vi "Locate HPRF Spark Laterally.vi"(5 "Ntheta":i32=16, 6 "Sensor Locations (cm)":dbl[][](array[numeric])=[[0.0, 0.0, -5.08], [11.43, 0.0, 0.0], [0.0, 11.43, 0.0], [-11.43, 0.0, 0.0], [0.0, -11.43, 0.0], [0.0, 0.0, 5.08]], 7 "Nr":i32=16, 8 "Sound Velocity (cm/s)":dbl=576000.0, 9 "Sampling Rate":i32=500000, 11 "Waveforms":dbl[][](array[numeric])) -> (2 "Coordinates (m)":cluster{"x":dbl, "y":dbl})   [LabVIEW 2013]
uses:
  <vilib>/Analysis/2dsp.llb/1D Cross Correlation (DBL).vi
  <vilib>/Analysis/NI_AALPro.lvlib
panel:
  out "Signals":dbl[][](graph)
  out "output variable 3":dbl
  out "output variable 2":dbl
  out "output variable":dbl
  out "subarray":dbl[][](array[numeric])
  out "size(s)":i32[](array[numeric])
  out "theta":dbl
  out "r":dbl
  out "Correlation":dbl[][](graph)
  out "Lag Matrix":dbl[][](array[numeric])
  # "Inputs"
  # "Output"
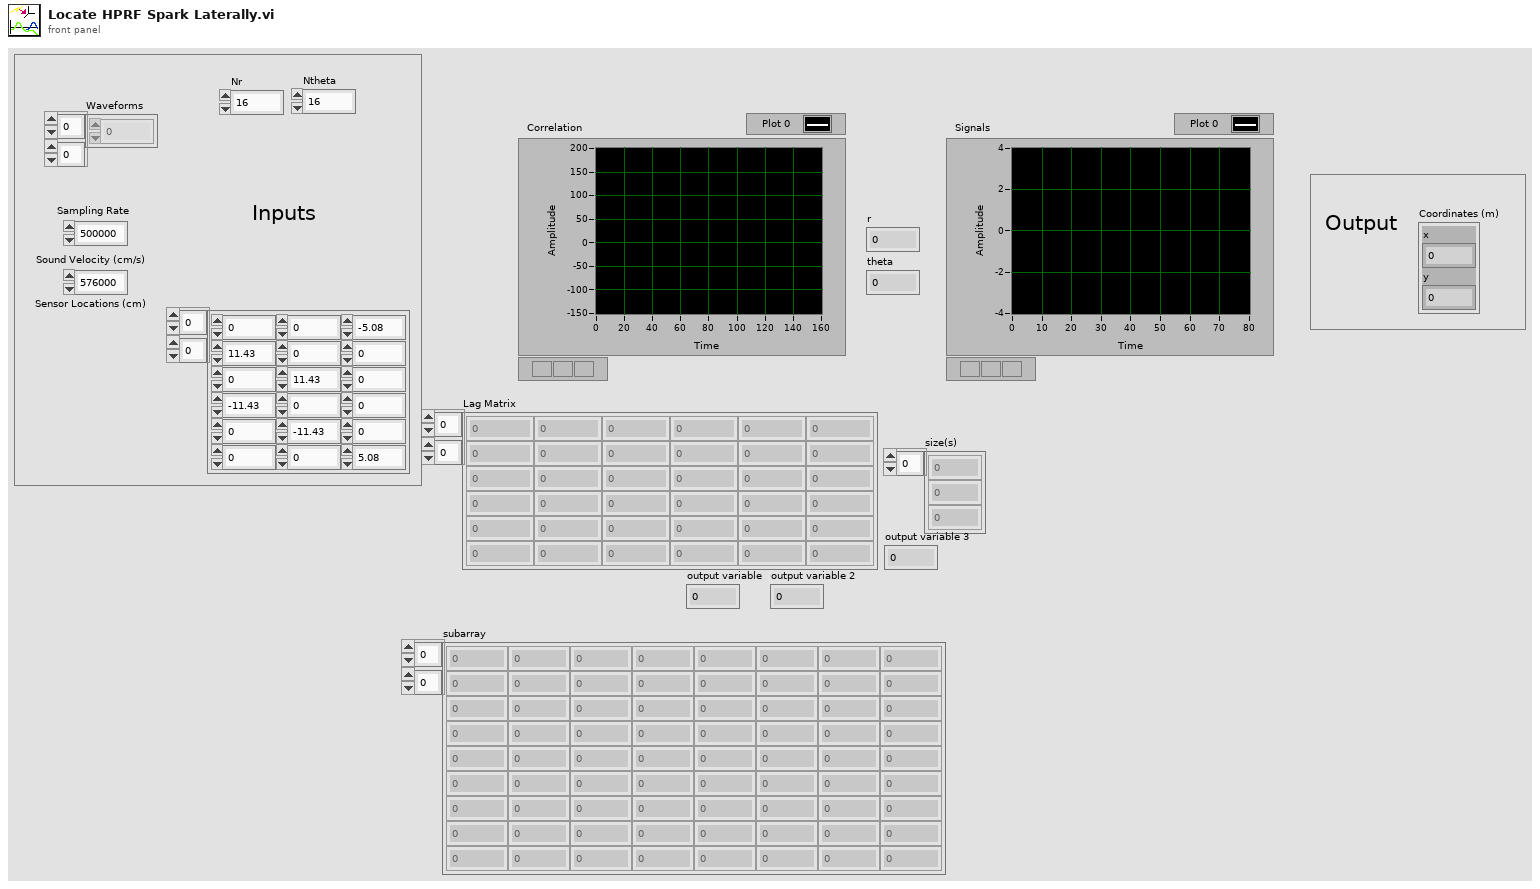
[diagram p1: front panel]
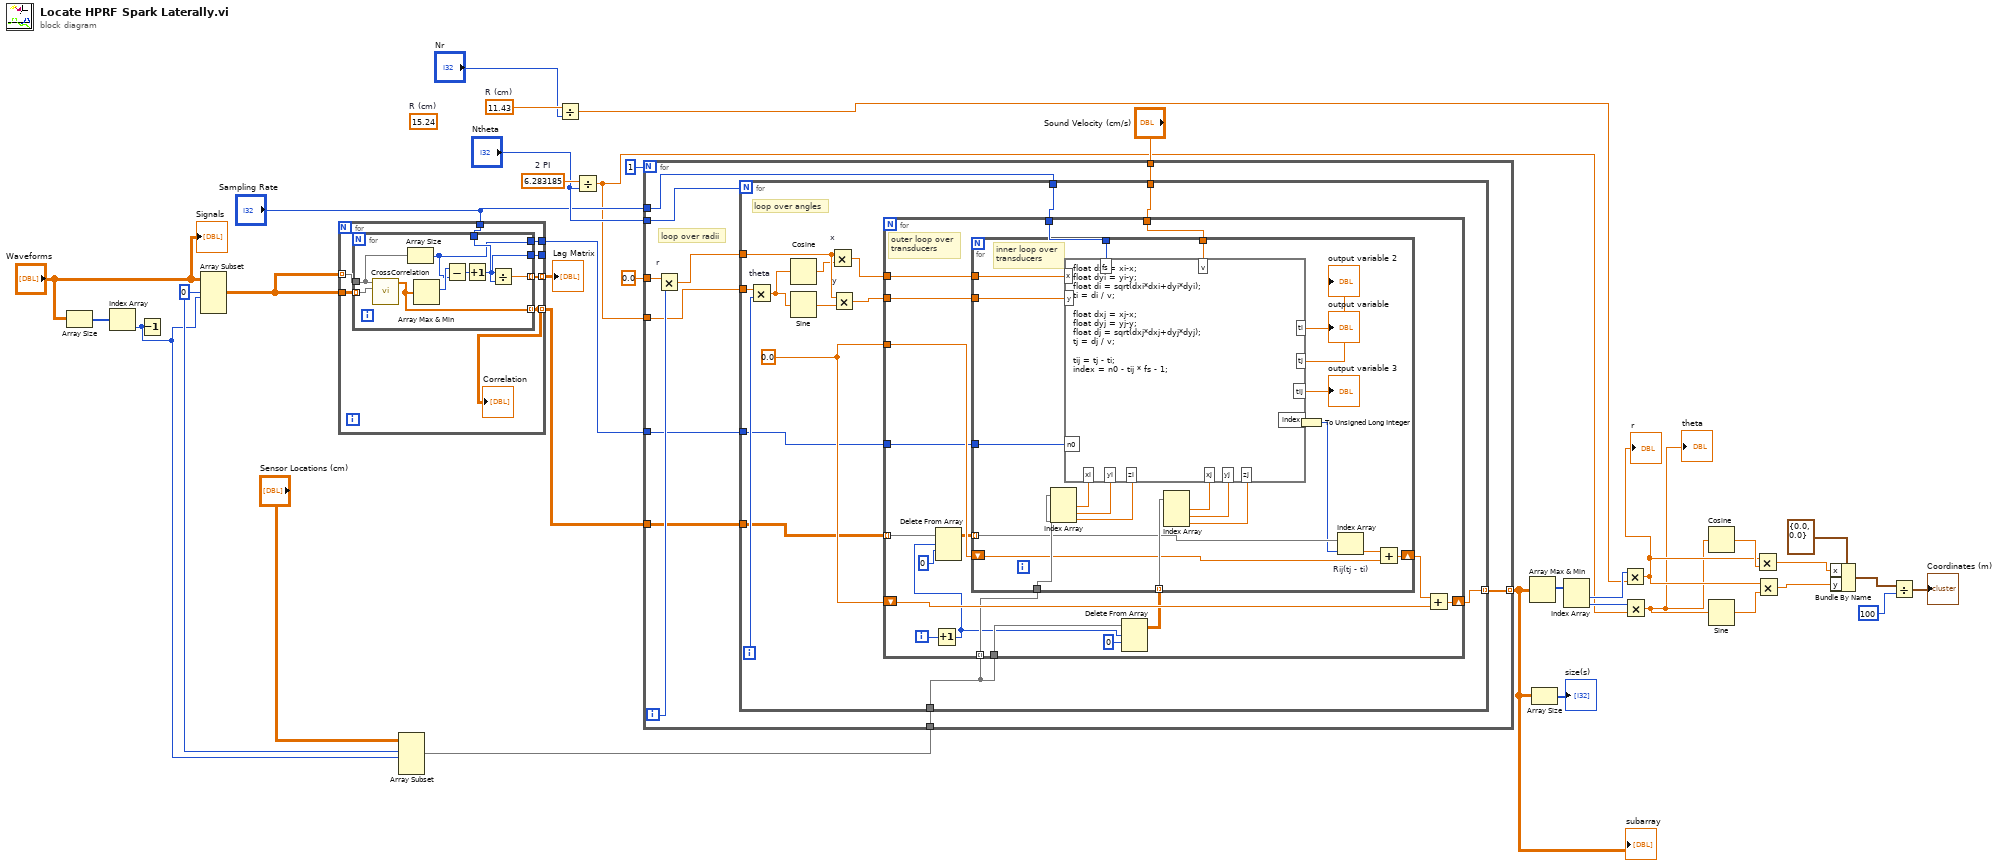
[diagram p0: block diagram]
diagram:
  (unwired) 15.24  # R (cm)
  w12 = 0 ("index")
  w34 = 11.43  # R (cm)
  w33 = 6.283185  # 2 PI
  n1 = Array Size(array="Waveforms") -> (size(s)=w8:i32[])
  n2 = Index Array(array=w8) -> (element=w6:i32)  [unwired: 1 in]
  n3 = Decrement(x=w6) -> ()  [unwired: 1 out]
  n4 = Array Subset(array="Waveforms", index (row)=w12, length (row)=w6) -> (w14:dbl[][])  [unwired: 2 in]
  n5 = for {
    tunnel: w14 -> [w41] mode=indexing
    tunnel: w14 -> [w42]
    tunnel: "Sampling Rate" -> [w40]
    tunnel: [w39] -> w35 mode=indexing
    tunnel: [w37] -> w29 mode=indexing
    tunnel: [w38] -> _
    tunnel: [w36] -> w5
    n6 = for {
      tunnel: w42 -> [w51] mode=indexing
      tunnel: w41 -> [w50]
      tunnel: w40 -> [w49]
      tunnel: [w48] -> w39 mode=indexing
      tunnel: [w45] -> w37 mode=indexing
      tunnel: [w46] -> w38
      tunnel: [w43] -> w36
      n7 = call-poly <vilib>:"CrossCorrelation.vi"("Y"=w51, "X"=w50) -> ("Rxy"=w45:dbl[])  [unwired: 8 in, 1 out]
      n8 = Array Size(array=w50) -> (size(s)=w43:i32)
      n9 = Array Max & Min(array=w45) -> (max index (indices)=w44:i32)  [unwired: 3 out]
      n10 = Subtract(x=w44, y=w43) -> (x-y=w47:i32)
      n11 = Increment(x=w47) -> (x+1=w46:i32)
      n12 = Divide(x=w46, y=w49) -> (x/y=w48:dbl)
    }
    "Correlation" <- w37
  }
  "Lag Matrix" <- w35
  n13 = Array Subset(array="Sensor Locations (cm)", index (row)=w12, length (row)=w6) -> (w9:dbl[][])  [unwired: 2 in]
  n14 = Divide(x=w34, y="Nr") -> (x/y=w25:dbl)
  n15 = Divide(x=w33, y="Ntheta") -> (x/y=w24:dbl)
  n16 = for {
    N: 1 -> [_]
    tunnel: [w62] -> w1 mode=indexing
    tunnel: "Ntheta" -> [w61]
    tunnel: 0.0 -> [w60]
    tunnel: w24 -> [w58]
    tunnel: w9 -> [w57]
    tunnel: "Sound Velocity (cm/s)" -> [w56]
    tunnel: "Sampling Rate" -> [w55]
    tunnel: w5 -> [w54]
    tunnel: w29 -> [w53]
    i -> [w59]
    # "loop over radii"
    n17 = Multiply "r"(x=w60, y=w59) -> (x*y=w52:dbl)
    n18 = for {
      N: w61 -> [_]
      tunnel: [w76] -> w62 mode=indexing
      tunnel: w58 -> [w75]
      tunnel: w52 -> [w73]
      tunnel: w57 -> [w70]
      tunnel: w56 -> [w69]
      tunnel: w55 -> [w68]
      tunnel: w54 -> [w67]
      tunnel: w53 -> [w66]
      i -> [w74]
      w77 = 0.0
      # "loop over angles"
      n19 = Multiply "theta"(x=w75, y=w74) -> (x*y=w65:dbl)
      n20 = Cosine(x=w65) -> (cos(x)=w72:dbl)
      n21 = Sine(x=w65) -> (sin(x)=w71:dbl)
      n22 = Multiply "x"(x=w73, y=w72) -> (x*y=w64:dbl)
      n23 = Multiply "y"(x=w73, y=w71) -> (x*y=w63:dbl)
      n24 = for {
        shift-right: [w92] -> w76
        shift-left: w77 -> [w93]
        tunnel: w77 -> [w95]
        tunnel: w64 -> [w91]
        tunnel: w63 -> [w90]
        tunnel: w70 -> [w89] mode=indexing
        tunnel: w70 -> [w84]
        tunnel: w69 -> [w88]
        tunnel: w68 -> [w87]
        tunnel: w67 -> [w86]
        tunnel: w66 -> [w81] mode=indexing
        i -> [w85]
        # "outer loop over\ntransducers"
        n25 = Increment(x=w85) -> (x+1=w78:i32)
        n26 = Delete From Array(array=w81, length=w78, index (row)=0) -> (array with subset deleted=w80:dbl[][])  [unwired: 1 in, 1 out]
        n27 = Delete From Array(array=w84, length=w78, index (row)=0) -> (array with subset deleted=w82:dbl[][])  [unwired: 1 in, 1 out]
        n28 = for {
          shift-right: [w103] -> w94
          shift-left: w95 -> [w101]
          tunnel: w91 -> [w114]
          tunnel: w90 -> [w113]
          tunnel: w82 -> [w116] mode=indexing
          tunnel: w89 -> [w117]
          tunnel: w88 -> [w115]
          tunnel: w87 -> [w108]
          tunnel: w86 -> [w107]
          tunnel: w80 -> [w105] mode=indexing
          # "inner loop over\ntransducers"
          n29 = Index Array(array=w117) -> (element #1=w112:dbl, element #2=w111:dbl, element #3=w100:dbl)  [unwired: 3 in]
          n30 = Index Array(array=w116) -> (element #1=w110:dbl, element #2=w109:dbl, element #3=w99:dbl)  [unwired: 3 in]
          n31 = formula code="float dxi = xi-x;\nfloat dyi = yi-y;\nfloat di = sqrt(dxi*dxi+dyi*dyi);\nti = di / v;\n\nfloat dxj = xj-x;\nfloat dyj = yj-y;\nfloat dj = sqrt(dxj*dxj+dyj*dyj);\ntj = dj / v;\n\ntij = tj - ti;\nindex = n0 - tij * fs - 1;"("xi"=w112, "yi"=w111, "xj"=w110, "yj"=w109, "x"=w114, "y"=w113, "v"=w115, "fs"=w108, "n0"=w107, "zi"=w100, "zj"=w99) -> ("index"=w106:dbl, "ti"=→"output variable":dbl, "tj"=→"output variable 2":dbl, "tij"=→"output variable 3":dbl)
          n32 = To Unsigned Long Integer(number=w106) -> (unsigned 32bit integer=w104:u32)
          n33 = Index Array "Rij(tj - ti)"(array=w105, index=w104) -> (element=w102:dbl)
          n34 = Add(x=w102, y=w101) -> (x+y=w103:dbl)
        }
        n35 = Add(x=w94, y=w93) -> (x+y=w92:dbl)
      }
    }
  }
  "subarray" <- w1
  n36 = Array Max & Min(array=w1) -> (max index (indices)=w28:i32[])  [unwired: 3 out]
  n37 = Array Size(array=w1) -> (size(s)=→"size(s)":i32[])
  n38 = Index Array(array=w28) -> (element #1=w27:i32, element #2=w26:i32)  [unwired: 2 in]
  n39 = Multiply(x=w27, y=w25) -> (x*y=w21:dbl)
  "r" <- w21
  n40 = Multiply(x=w26, y=w24) -> (x*y=w20:dbl)
  "theta" <- w20
  n41 = Cosine(x=w20) -> (cos(x)=w23:dbl)
  n42 = Sine(x=w20) -> (sin(x)=w22:dbl)
  n43 = Multiply ("x*y")(x=w21, y=w23) -> (x*y=w19:dbl)
  n44 = Multiply ("x*y")(x=w21, y=w22) -> (x*y=w18:dbl)
  n45 = Bundle By Name(cluster=cluster{"x":dbl, "y":dbl} {"x"=0.0, "y"=0.0} ("input cluster"), "x"=w19, "y"=w18) -> (w16:cluster{"x":dbl, "y":dbl})
  n46 = Divide(x=w16, y=100 ("index (row)")) -> (x/y=→"Coordinates (m)":cluster{"x":dbl, "y":dbl})
  "Signals" <- "Waveforms"
